vi "ni_move.vi"(6 "Axis enable":bool[](array[boolean])=[TRUE, TRUE, TRUE, TRUE], 7 "Timeout":u32=60000, 8 "error in":errorcluster, 9 "Axis positions":dbl[](array[numeric])=[0.0, 0.0, 0.0, 0.0], 10 "Absolute":bool=TRUE) -> (0 "error out":errorcluster)   [LabVIEW 2014]
uses:
  <vilib>/Motion/FlexMotion/CustomControls/CustomControls.llb/AxisOrVectorSpaceControl To Control.flx
  <vilib>/Motion/FlexMotion/CustomControls/CustomControls.llb/AxisOrVectorSpace To Configure.flx
  <vilib>/Motion/FlexMotion/FunctionsVIs/StartStopMotion.llb/Start Motion (8 axes).flx
  <vilib>/Motion/FlexMotion/FunctionsVIs/Trajectory.llb/Wait for Move Complete (8 axes).flx
panel:
  # "The purposes of axis enable is to allow a subset of axes to be driven in absolute position mode without changing (or knowing) the positions of the other axes.   Being disabled just means that we don't want to move that axis, not that we want it powered down."
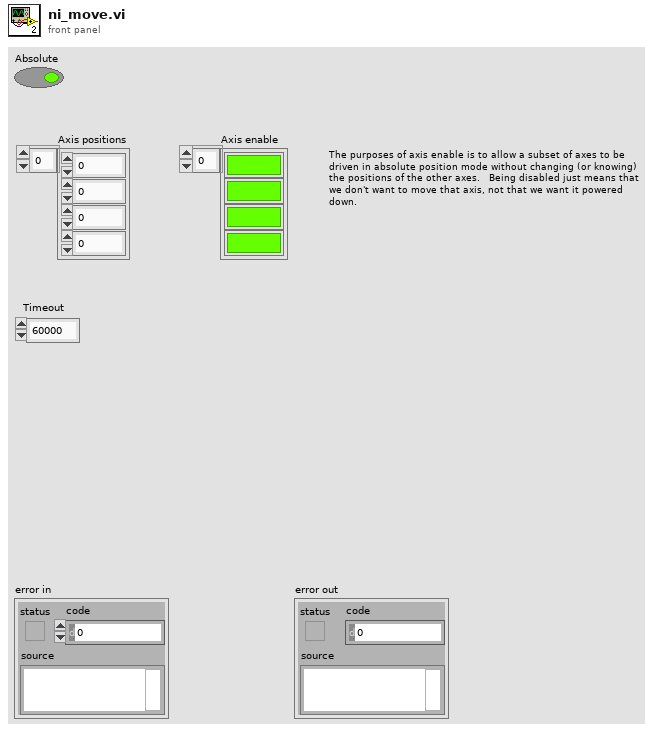
[diagram p1: front panel]
types:
  T1 = typedef "Board Id" = u8
  T2 = enum16{"Absolute Position", "Relative Position", "Velocity", "Relative to Cap Pos", "Modulus Position", "Absolute Contouring", "Relative Contouring"}
  T3 = typedef "AxisOrVectorSpaceControl To Control.flx" = u16
  T4 = typedef "AxisOrVectorSpace To Configure.flx" = u16
  T5 = typedef "Resource Out (Enum).flx" = u16
  T6 = typedef "Bd Id Out" = u8
  T7 = cluster{"Axis enable[0]":bool, "Axis enable[1]":bool, "Axis enable[2]":bool, "Axis enable[3]":bool, "Axis enable[4]":bool, "Axis enable[5]":bool, "Axis enable[6]":bool, "Axis enable[7]":bool}
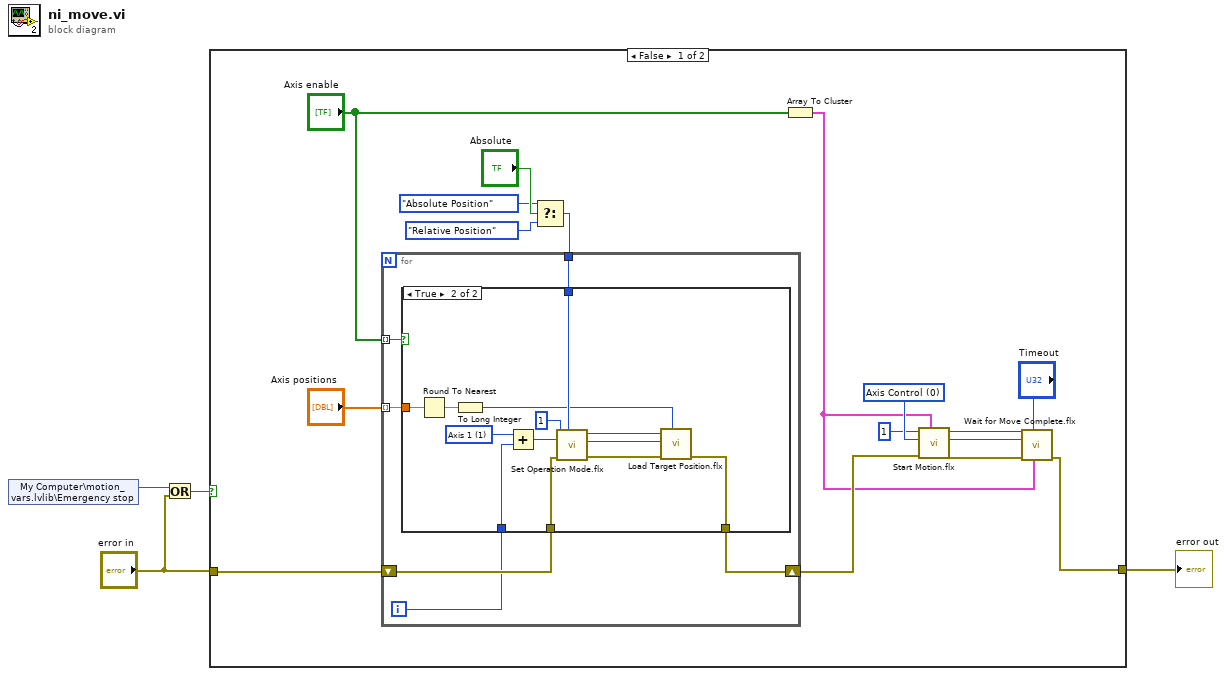
[diagram p0: block diagram]
diagram:
  n1 = shared-variable "My Computer\\motion_vars.lvlib\\Emergency stop"() -> (w3:bool)  [unwired: 1 in, 1 out]
  n2 = Or(x=w3, y="error in") -> (x .or. y?=w1:bool)
  n3 = case shown="False" w1 {
    tunnel: "error in" -> [w19 w41]
    tunnel: [w8 w41] -> w4
    frame False {
      w12 = T3 0 items=["Axis Control"=0, "Axis 1"=1, "Axis 2"=2, "Axis 3"=3, "Axis 4"=4, "Axis 5"=5, "Axis 6"=6, "Axis 7"=7, "Axis 8"=8, "Vector Space Control"=16, "Vector Space 1"=17, "Vector Space 2"=18, "Vector Space 3"=19, "Vector Space 4"=20] ("Axis or Vector Space")
      n4 = Select(t=T2."Absolute Position" ("Position Mode (Absolute)"), s="Absolute", f=T2."Relative Position" ("Position Mode (Absolute)")) -> (s? t:f=w16:T2)
      n5 = for {
        tunnel: "Axis enable" -> [w24] mode=indexing
        tunnel: "Axis positions" -> [w23] mode=indexing
        shift-right: [w22] -> w13
        shift-left: w19 -> [w26]
        tunnel: w16 -> [w25]
        i -> [w21]
        n6 = case shown="True" w24 {
          tunnel: w26 -> [w27 w38]
          tunnel: w21 -> [_ w37]
          tunnel: w25 -> [_ w36]
          tunnel: w23 -> [_ w32]
          tunnel: [w27 w29] -> w22
          frame False {
          }
          frame True {
            w40 = T4 1 items=["Axis 1"=1, "Axis 2"=2, "Axis 3"=3, "Axis 4"=4, "Axis 5"=5, "Axis 6"=6, "Axis 7"=7, "Axis 8"=8, "Vector Space 1"=17, "Vector Space 2"=18, "Vector Space 3"=19, "Vector Space 4"=20] ("Axis or Vector Space")
            n7 = Round To Nearest(number=w32) -> (nearest integer value=w31:dbl)
            n8 = To Long Integer(number=w31) -> (32bit integer=w30:i32)
            n9 = Add(x=w40, y=w37) -> (x+y=w39:i32)
            n10 = call <vilib>:"Set Operation Mode.flx"("Position Mode (Absolute)"=w36, "error in (no error)"=w38, "Axis or Vector Space"=w39, "Board ID"=T1 1) -> ("error out"=w33:errorcluster, "Resource Output"=w34:T5, "Bd ID Out"=w35:T6)  [unwired: 2 in]
            n11 = call <vilib>:"Load Target Position.flx"("Target Position (0)"=w30, "error in (no error)"=w33, "Axis"=w34, "Board ID"=w35) -> ("error out"=w29:errorcluster)  [unwired: 3 in, 2 out]
          }
        }
      }
      n12 = Array To Cluster(array="Axis enable") -> (cluster=w11:T7)
      n13 = call-poly <vilib>:"Start Motion.flx"("Axis/VS Map (Disabled)"=w11, "error in (no error)"=w13, "Axis or Vector Space"=w12, "Board ID"=T1 1) -> ("error out"=w9:errorcluster, "Resource Output"=w10:T5, "Bd ID Out"=w6:T6)  [unwired: 2 in]
      n14 = call-poly <vilib>:"Wait for Move Complete.flx"("Axis/VS Map (Disabled)"=w11, "Timeout (10000 ms)"="Timeout", "error in (no error)"=w9, "Axis or Vector Space"=w10, "Board ID"=w6) -> ("error out"=w8:errorcluster)  [unwired: 3 in, 3 out]
    }
    frame True {
    }
  }
  "error out" <- w4
